vi "Swerve Drive Visuals.vi"(10 "Pod Setpoints (ft/s and deg)":T8, 11 "Motors":T1) -> (2 "Swerve Visualizer":cluster{dbl[], dbl[]}[](graph), 3 "Pod Comparisons (Diff -> Setpoint - Actual)":T9)   [LabVIEW 2020]
uses:
  swerve/ctl/Pod Setpoints.ctl
  swerve/ctl/Swerve Motors.ctl
  swerve/ctl/4 Motor Set.ctl
  <vilib>/Rock Robotics/WPI/MotorControl/WPI_MotorControlDeviceRef.ctl
  <vilib>/Rock Robotics/WPI/MotorControl/WPI_MotorControlType.ctl
  <vilib>/Rock Robotics/SystemInterfaces/DIO/FPGA_DIOPWMChannel.ctl
  <vilib>/Rock Robotics/WPI/PWM/WPI_PWMDeadband.ctl
  <vilib>/Rock Robotics/SystemInterfaces/DIO/FPGA_DIOChannel.ctl
  <vilib>/Analysis/coordinate.llb/Angle Range (Degree).ctl
  <vilib>/Analysis/coordinate.llb/Angle Units.ctl
  <vilib>/Analysis/coordinate.llb/Wrap Angle (array).vi
  <vilib>/Analysis/NI_AAL_Angle.lvlib
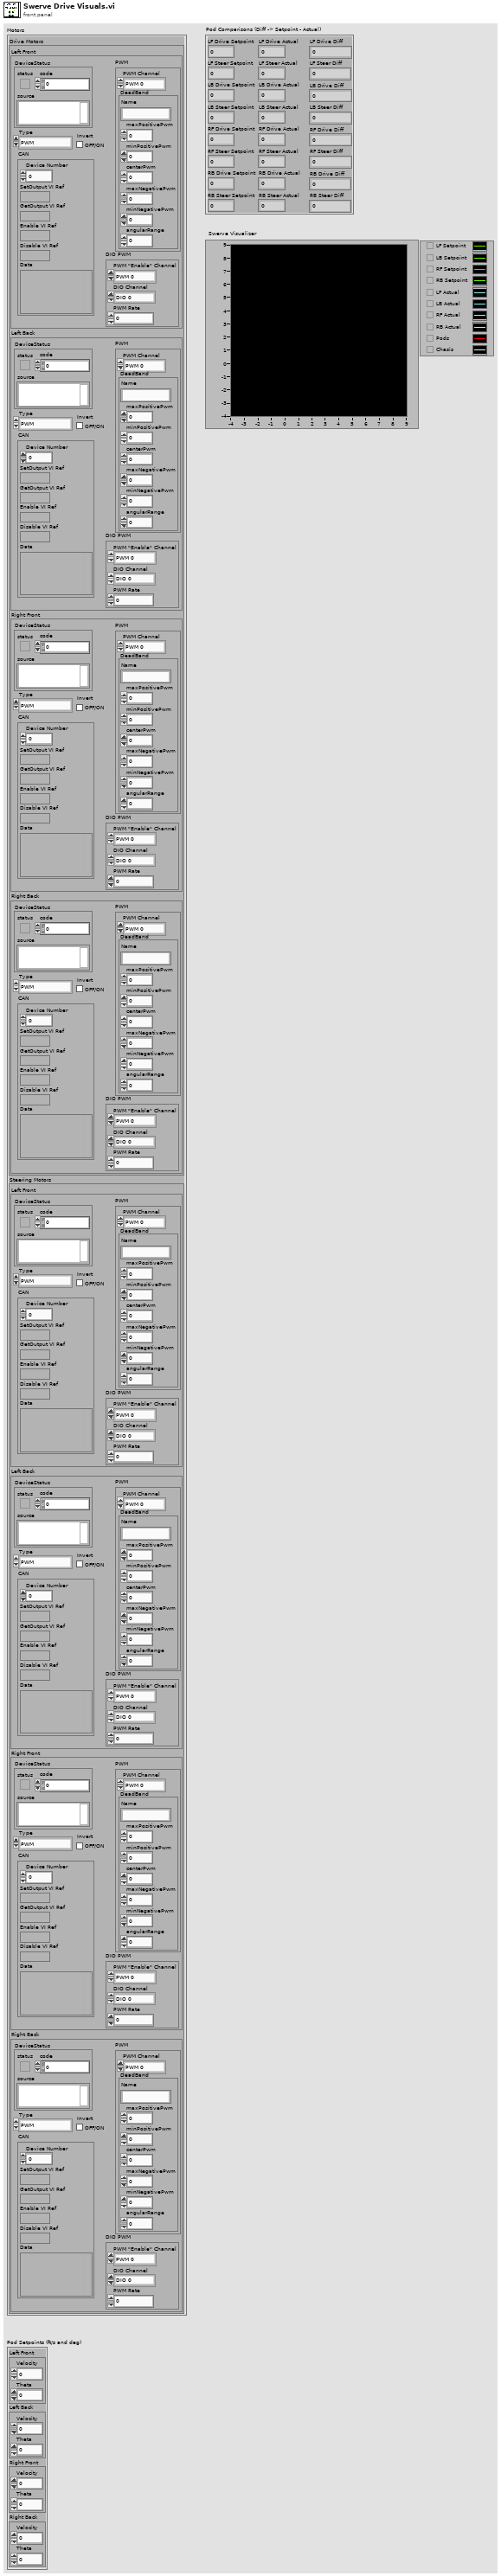
[diagram p1: front panel]
types:
  T1 = typedef "Swerve Motors.ctl" = cluster{"Drive Motors":T2, "Steering Motors":T2}
  T2 = typedef "4 Motor Set.ctl" = cluster{"Left Front":T3, "Left Back":T3, "Right Front":T3, "Right Back":T3}
  T3 = typedef "WPI_MotorControlDeviceRef.ctl" = cluster{"DeviceStatus":errorcluster, "Type":T4, "PWM":cluster{"PWM Channel":T5, "DeadBand":T6}, "CAN":cluster{"Device Number":u8, "SetOutput VI Ref":variant, "GetOutput VI Ref":variant, "Enable VI Ref":variant, "Disable VI Ref":variant, "Data":variant}, "Invert":bool, "DIO PWM":cluster{"PWM \"Enable\" Channel":T5, "DIOChannel":T7, "PWM Rate":dbl}}
  T4 = typedef "WPI_MotorControlType.ctl" = enum16{"PWM", "CAN", "DIO PWM"}
  T5 = typedef "FPGA_DIOPWMChannel.ctl" = enum8{"PWM 0", "PWM 1", "PWM 2", "PWM 3", "PWM 4", "PWM 5", "PWM 6", "PWM 7", "PWM 8", "PWM 9", "PWM MXP 0", "PWM MXP 1", "PWM MXP 2", "PWM MXP 3", "PWM MXP 4", "PWM MXP 5", "PWM MXP 6", "PWM MXP 7", "PWM MXP 8", "PWM MXP 9", "Invalid"}
  T6 = typedef "WPI_PWMDeadband.ctl" = cluster{"Name":string, "maxPositivePwm":i32, "minPositivePwm":i32, "centerPwm":i32, "maxNegativePwm":i32, "minNegativePwm":i32, "angularRange":u16}
  T7 = typedef "FPGA_DIOChannel.ctl" = enum8{"DIO 0", "DIO 1", "DIO 2", "DIO 3", "DIO 4", "DIO 5", "DIO 6", "DIO 7", "DIO 8", "DIO 9", "DIO MXP 0", "DIO MXP 1", "DIO MXP 2", "DIO MXP 3", "DIO MXP 4", "DIO MXP 5", "DIO MXP 6", "DIO MXP 7", "DIO MXP 8", "DIO MXP 9", "DIO MXP 10", "DIO MXP 11", "DIO MXP 12", "DIO MXP 13", "DIO MXP 14", "DIO MXP 15", "SPI Port CS1", "SPI Port CS2", "SPI Port CS3", "SPI Port MISO", "SPI Port MOSI", "Invalid"}
  T8 = typedef "Pod Setpoints.ctl" = cluster{"Left Front":cluster{"Velocity":dbl, "Theta":dbl}, "Left Back":cluster{"Velocity":dbl, "Theta":dbl}, "Right Front":cluster{"Velocity":dbl, "Theta":dbl}, "Right Back":cluster{"Velocity":dbl, "Theta":dbl}}
  T9 = cluster{"LF Drive Setpoint":dbl, "LF Steer Setpoint":dbl, "LB Drive Setpoint":dbl, "LB Steer Setpoint":dbl, "RF Drive Setpoint":dbl, "RF Steer Setpoint":dbl, "RB Drive Setpoint":dbl, "RB Steer Setpoint":dbl, "LF Drive Actual":dbl, "LF Steer Actual":dbl, "LB Drive Actual":dbl, "LB Steer Actual":dbl, "RF Drive Actual":dbl, "RF Steer Actual":dbl, "RB Drive Actual":dbl, "RB Steer Actual":dbl, "LF Drive Diff":dbl, "LF Steer Diff":dbl, "LB Drive Diff":dbl, "LB Steer Diff":dbl, "RF Drive Diff":dbl, "RF Steer Diff":dbl, "RB Drive Diff":dbl, "RB Steer Diff":dbl}
  T10 = typedef "NI_AAL_Angle.lvlib/Angle Units.ctl" = i32
  T11 = typedef "NI_AAL_Angle.lvlib/Angle Range (Degree).ctl" = u16
  T12 = cluster{"Left Front":dbl, "Left Back":dbl, "Right Front":dbl, "Right Back":dbl}
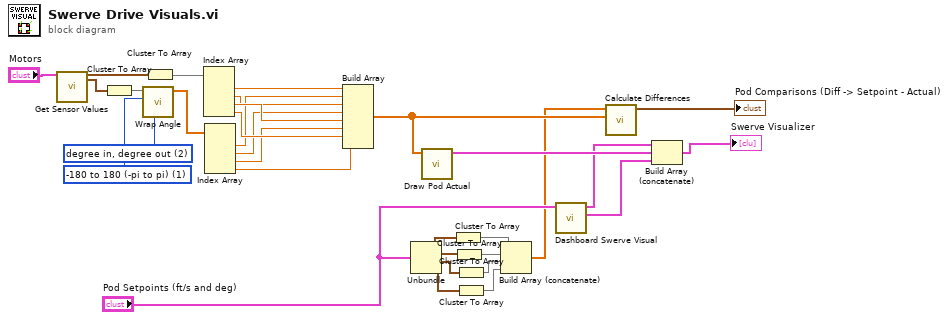
[diagram p0: block diagram]
diagram:
  w21 = T10 2 items=["radian in, radian out", "radian in, degree out", "degree in, degree out", "degree in, radian out"] ("angle units")
  w20 = T11 1 items=["none", "-180 to 180 (-pi to pi)", "0 to 360 (0 to 2pi)"] ("angle range")
  n1 = call "Get Sensor Values.vi"("Motors"="Motors") -> ("Drive Velocities (ft/s)"=w29:T12, "Steer Angles (degrees)"=w30:T12)  [unwired: 13 in, 4 out]
  n2 = Cluster To Array(cluster=w30) -> (array=w18:dbl[])
  n3 = call-poly <vilib>:"Wrap Angle.vi"("angle units"=w21, "angle range"=w20, "Angle In"=w18) -> ("Angle Out"=w19:dbl[])  [unwired: 7 in, 1 out]
  n4 = Cluster To Array(cluster=w29) -> (array=w9:dbl[])
  n5 = Index Array(array=w9) -> (element #1=w10:dbl, element #2=w12:dbl, element #3=w14:dbl, element #4=w16:dbl)  [unwired: 4 in]
  n6 = Index Array(array=w19) -> (element #1=w11:dbl, element #2=w13:dbl, element #3=w15:dbl, element #4=w17:dbl)  [unwired: 4 in]
  n7 = Build Array(w10, w11, w12, w13, w14, w15, w16, w17) -> (w23:dbl[])
  n8 = Unbundle("Pod Setpoints (ft/s and deg)") -> ("Left Front"=w1:cluster{"Velocity":dbl, "Theta":dbl}, "Left Back"=w2:cluster{"Velocity":dbl, "Theta":dbl}, "Right Front"=w3:cluster{"Velocity":dbl, "Theta":dbl}, "Right Back"=w4:cluster{"Velocity":dbl, "Theta":dbl})
  n9 = call "Draw Pod Actual.vi"("Pod Sensor Readings"=w23) -> ("Actual Pod Vectors"=w26:cluster{dbl[], dbl[]}[])  [unwired: 10 in]
  n10 = Cluster To Array(cluster=w1) -> (array=w5:dbl[])
  n11 = Cluster To Array(cluster=w2) -> (array=w6:dbl[])
  n12 = Cluster To Array(cluster=w3) -> (array=w7:dbl[])
  n13 = Cluster To Array(cluster=w4) -> (array=w8:dbl[])
  n14 = Build Array (concatenate)(w5, w6, w7, w8) -> (w22:dbl[])
  n15 = call "Dashboard Swerve Visual.vi"("Pod Setpoints (ft/s and deg)"="Pod Setpoints (ft/s and deg)") -> ("Robot"=w27:cluster{dbl[], dbl[]}[], "Pod Vectors"=w25:cluster{dbl[], dbl[]}[])  [unwired: 9 in]
  n16 = call "Calculate Differences.vi"("Actual"=w23, "Setpoint"=w22) -> ("Pod Comparisons (Diff -> Setpoint - Actual)"=→"Pod Comparisons (Diff -> Setpoint - Actual)":T9)  [unwired: 9 in]
  n17 = Build Array (concatenate)(w25, w26, w27) -> (→"Swerve Visualizer":cluster{dbl[], dbl[]}[])
